vi "Report Conditions.vi"(11 "Sequence Config in":refnum<class "Sequence Config.lvclass">) -> (2 "Report Conditions":bool, 3 "Sequence Config out":refnum<class "Sequence Config.lvclass">)   [LabVIEW 2023, in "VolatusSeqConfig.lvlib" / "Sequence Config.lvclass"]
uses:
  Sequence Config.lvclass
  Sequence Config.lvclass/Sequence Config.ctl
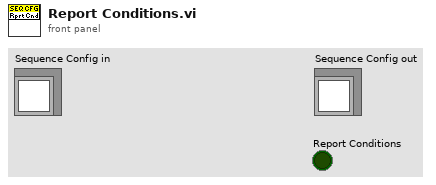
[diagram p1: front panel]
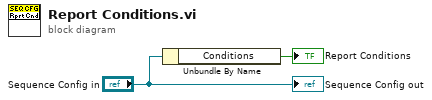
[diagram p0: block diagram]
diagram:
  n1 = Unbundle By Name("Sequence Config in") -> ("Conditions"=→"Report Conditions":bool)
  "Sequence Config out" <- "Sequence Config in"
